vi "AC_Dummy.vi"(0 "Top":string, 1 "UL":string, 7 "ML":dbl, 9 "4":dbl, 10 "5":dbl, 12 "3":dbl, 13 "BRM":dbl, 14 "TRM 2":dbl, 15 "2":dbl, 18 "1":dbl, 19 "Error In":errorcluster) -> (4 "UR":string, 5 "MR":i32, 6 "Error Out":errorcluster)   [LabVIEW 2011]
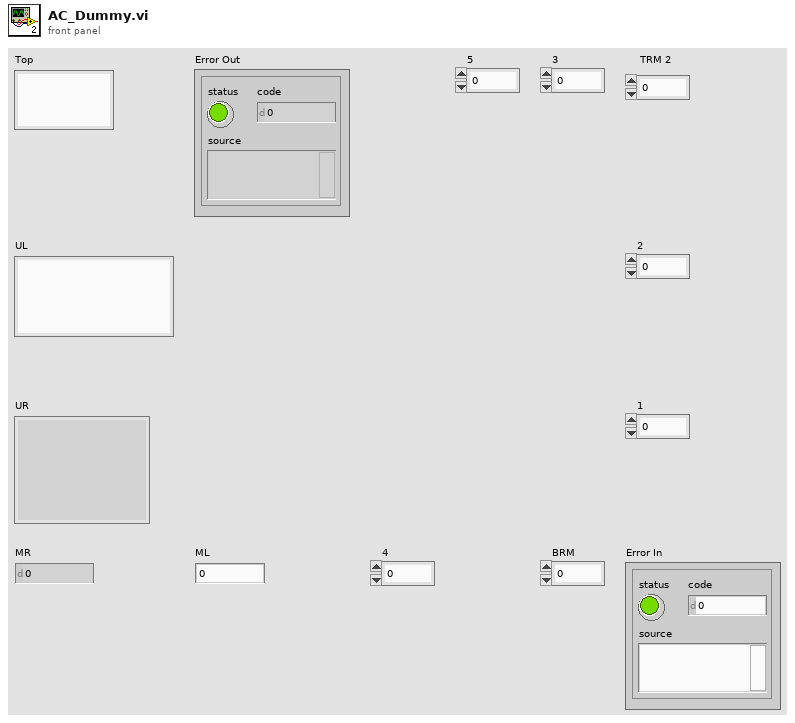
[diagram p1: front panel]
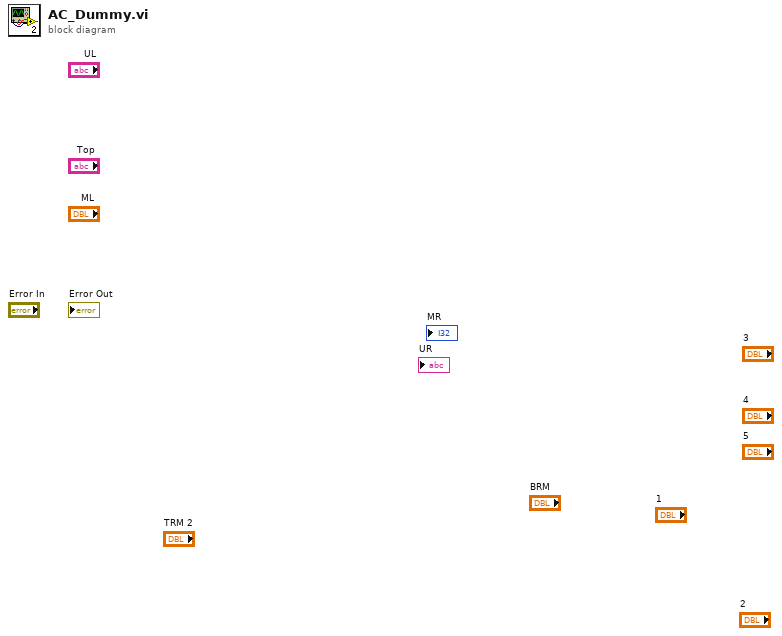
[diagram p0: block diagram]
diagram:
